vi "Parse Cmds.vi"(11 "Command List":T1) -> ()   [LabVIEW 2015]
uses:
  IntakeController/Typedef/Command List.ctl
  Typedef/IntakeControllerActions.ctl
  IntakeController/Typedef/Front Arm List.ctl
  IntakeController/Typedef/Rear Arm List.ctl
  Typedef/IntakeControllerMsg.ctl
  ArmController/ArmController.lvlib
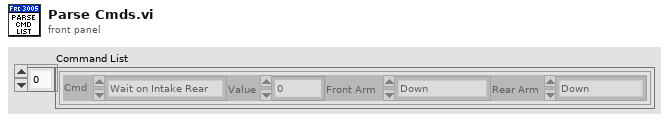
[diagram p1: front panel]
types:
  T1 = typedef "Command List.ctl" = cluster{"Cmd":T2, "Value":dbl, "Front Arm":T3, "Rear Arm":T4}[]
  T2 = typedef "IntakeControllerActions.ctl" = enum16{"Wait on Intake Rear", "Wait on Angle Rear", "Go To Angle Rear", "Wait on Intake Front", "Wait on Angle Front", "Set Roller Front", "Set Roller Rear", "Go To Angle Front", "Wait ms"}
  T3 = typedef "Front Arm List.ctl" = enum16{"Down", "Pickup", "Shoot", "Turtle", "Intake Transfer", "Extra1", "Extra2"}
  T4 = typedef "Rear Arm List.ctl" = enum16{"Down", "Pickup", "Shoot", "Turtle", "Intake Block", "Intake Transfer", "Extra1", "Extra2"}
  T5 = cluster{"Down":dbl, "Pickup":dbl, "Shoot":dbl, "Turtle":dbl, "Intake Block":dbl, "Intake Transfer":dbl}
  T6 = cluster{"Down":dbl, "Pickup":dbl, "Shoot":dbl, "Turtle":dbl, "Intake Transfer":dbl}
  T7 = typedef "IntakeControllerMsg.ctl" = cluster{"Cmd":T2, "Data":variant}
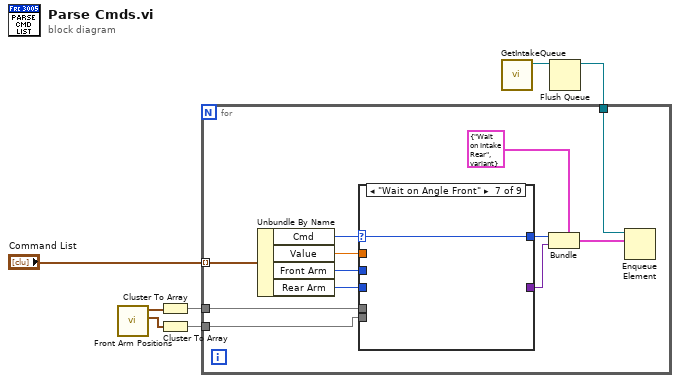
[diagram p0: block diagram]
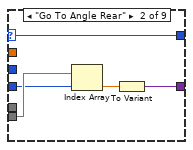
[diagram p3: hidden frame]
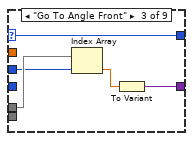
[diagram p4: hidden frame]
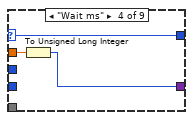
[diagram p5: hidden frame]
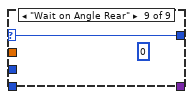
[diagram p9: hidden frame]
diagram:
  n1 = call "Front Arm Positions.vi"() -> ("Rear Arm"=w5:T5, "Front Arm"=w4:T6)  [unwired: 10 in]
  n2 = Cluster To Array(cluster=w4) -> (array=w6:dbl[])
  n3 = Cluster To Array(cluster=w5) -> (array=w7:dbl[])
  n4 = call "GetIntakeQueue.vi"() -> ("queue out"=w1:refnum<queue>)  [unwired: 11 in]
  n5 = Flush Queue(queue=w1) -> (queue out=w3:refnum<queue>)  [unwired: 1 in, 2 out]
  n6 = for {
    tunnel: "Command List" -> [w18] mode=indexing
    tunnel: w3 -> [w15]
    tunnel: w6 -> [w13]
    tunnel: w7 -> [w14]
    n7 = Unbundle By Name(w18) -> ("Cmd"=w17:T2, "Value"=w9:dbl, "Front Arm"=w10:T3, "Rear Arm"=w12:T4)
    n8 = case shown="\"Wait on Angle Front\"" w17 {
      selector: w17 -> [w20 w25 w30 w33 w35 w37 w38 w39 w40]
      tunnel: [w20 w25 w30 w33 w35 w37 w38 w39 w40] -> w16
      tunnel: w14 -> [_ w24 _ _ _ _ _ _ _]
      tunnel: w13 -> [_ _ w27 _ _ _ _ _ _]
      tunnel: w12 -> [_ w23 _ _ _ _ _ _ _]
      tunnel: [_ w21 w28 w31 w34 w36 _ _ _] -> w11
      tunnel: w10 -> [_ _ w26 _ _ _ _ _ _]
      tunnel: w9 -> [_ _ _ w32 w34 w36 _ _ _]
      frame "Wait on Intake Rear" {
      }
      frame "Go To Angle Rear" {
        n9 = Index Array(array=w24, index=w23) -> (element=w22:dbl)
        n10 = To Variant(anything=w22) -> (Variant=w21:variant)
      }
      frame "Go To Angle Front" {
        n11 = Index Array(array=w27, index=w26) -> (element=w29:dbl)
        n12 = To Variant(anything=w29) -> (Variant=w28:variant)
      }
      frame "Wait ms" {
        n13 = To Unsigned Long Integer(number=w32) -> (unsigned 32bit integer=w31:u32)
      }
      frame "Set Roller Front" {
      }
      frame "Set Roller Rear" {
      }
      frame "Wait on Angle Front" {
      }
      frame "Wait on Intake Front" {
      }
      frame "Wait on Angle Rear" {
        (unwired) 0
      }
    }
    n14 = Bundle(cluster=T7 {"Cmd"=enum."Wait on Intake Rear", "Data"=variant} ("element"), "Cmd"=w16, "Data"=w11) -> (w8:T7)
    n15 = Enqueue Element(queue=w15, element=w8) -> ()  [unwired: 2 in, 3 out]
  }
